vi "FTW-TransferClient-Download.vi"(0 "Transfer Client":refnum<k24>, 5 "Remote URI":string, 11 "error in":errorcluster) -> (4 "Transfer Client out":refnum<k24>, 6 "Data":string, 8 "Elapsed Time":dbl format="%.4psec", 15 "error out":errorcluster)   [LabVIEW 2014]
panel:
  # "Inputs"
  # "Outputs"
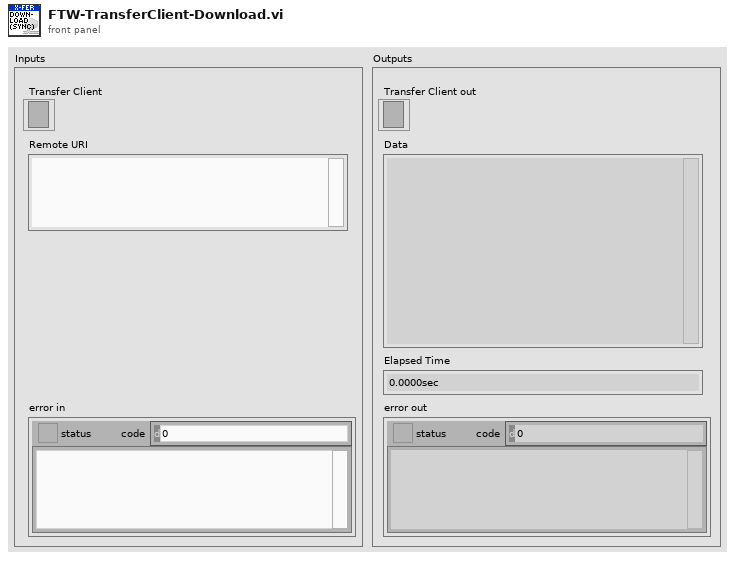
[diagram p1: front panel]
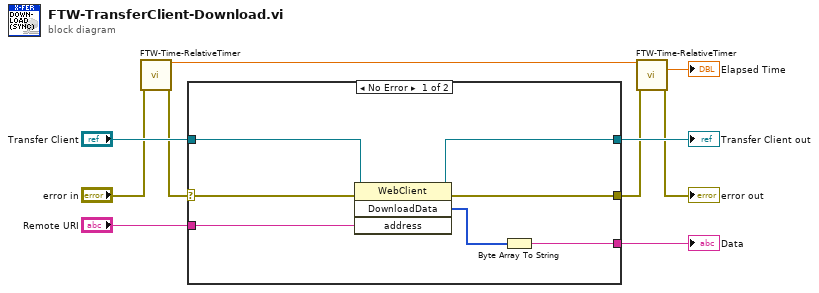
[diagram p0: block diagram]
diagram:
  n1 = call "FTW-Time-RelativeTimer.vi"("error in"="error in") -> ("Current Timer Value"=w3:dbl, "error out"=w6:errorcluster)  [unwired: 12 in, 1 out]
  n2 = case shown="No Error" w6 {
    selector: w6 -> [w14 w18]
    tunnel: "Transfer Client" -> [w13 w19]
    tunnel: [w16 _] -> w9
    tunnel: [w15 w18] -> w4
    tunnel: [w12 w19] -> w8
    tunnel: "Remote URI" -> [w11 _]
    frame No Error {
      n3 = invoke class="WebClient" method="DownloadData"(reference=w13, error in=w14, "address"=w11) -> (reference out=w12:refnum<k24>, error out=w15:errorcluster, "DownloadData"=w17:u8[])  [unwired: 1 in, 1 out]
      n4 = Byte Array To String(unsigned byte array=w17) -> (string=w16:string)
    }
    frame Error {
    }
  }
  "Transfer Client out" <- w8
  "Data" <- w9
  n5 = call "FTW-Time-RelativeTimer.vi"("Previous Timer Value"=w3, "error in"=w4) -> ("Elapsed Time"=→"Elapsed Time":dbl, "error out"=→"error out":errorcluster)  [unwired: 11 in, 1 out]
